vi "Minimize Polymer.vi"(8 "Error In":errorcluster, 11 "Unreacted Polymer":string) -> (0 "Error Out":errorcluster, 1 "Size of Redux Polymer":i32, 2 "Redux Polymer":string, 3 "Redux Element":string)   [LabVIEW 2019]
doc: "Produce the smallest polymer possible by removing a single element, then reacting the polymer as normal."
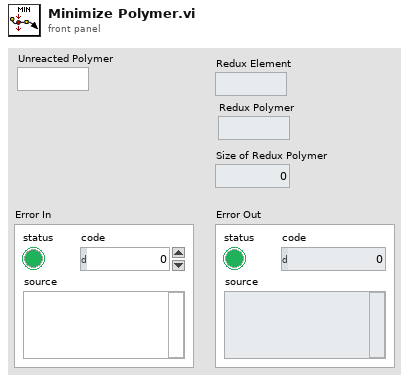
[diagram p1: front panel]
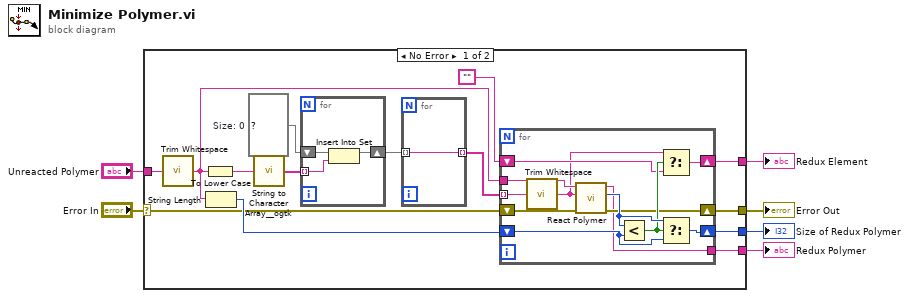
[diagram p0: block diagram]
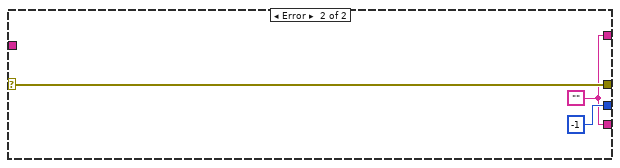
[diagram p2: hidden frame]
diagram:
  n1 = case shown="No Error" "Error In" {
    selector: "Error In" -> [w13 w38]
    tunnel: [w20 -1 ("Size of Polymer")] -> w6
    tunnel: [w19 w37] -> w5
    tunnel: "Unreacted Polymer" -> [w11 _]
    tunnel: [w12 w38] -> w2
    tunnel: [w7 w37] -> w1
    frame No Error {
      w16 = set{string} {}  # Size: 0
      n2 = call <vilib>:"Trim Whitespace.vi"("string"=w11) -> ("trimmed string"=w10:string)  [unwired: 1 in]
      n3 = To Lower Case(string=w10) -> (all lower case string=w14:string)
      n4 = String Length(string=w10) -> (length=w17:i32)
      n5 = call <userlib>:"String to Character Array__ogtk.vi"("Input String"=w14) -> ("Character Array"=w15:string[])
      n6 = for {
        tunnel: w15 -> [w35] mode=indexing
        shift-right: [w34] -> w9
        shift-left: w16 -> [w36]
        n7 = Insert Into Set(10:w35, 11:w36) -> (3:w34:set{string})  [unwired: 1 out]
      }
      n8 = for {
        tunnel: [w21] -> w8 mode=indexing
        tunnel: w9 -> [w21] mode=indexing
      }
      n9 = for {
        tunnel: w10 -> [w33]
        shift-right: [w30] -> w20
        shift-left: w17 -> [w31]
        shift-right: [w27] -> w19
        shift-left: "" -> [w28]
        shift-right: [w26] -> w12
        shift-left: w13 -> [w25]
        tunnel: w8 -> [w24] mode=indexing
        tunnel: [w22] -> w7
        n10 = call <vilib>:"Trim Whitespace.vi"("string"=w24) -> ("trimmed string"=w23:string)  [unwired: 1 in]
        n11 = call "React Polymer.vi"("Error In"=w25, "Redux Element"=w23, "Unreacted Polymer"=w33) -> ("Error Out"=w26:errorcluster, "Size of Polymer"=w32:i32, "Polymer"=w22:string)  [unwired: 6 in]
        n12 = Less?(x=w32, y=w31) -> (x < y?=w29:bool)
        n13 = Select(t=w23, s=w29, f=w28) -> (s? t:f=w27:string)
        n14 = Select(t=w32, s=w29, f=w31) -> (s? t:f=w30:i32)
      }
    }
    frame Error {
      w37 = ""
    }
  }
  "Size of Redux Polymer" <- w6
  "Redux Element" <- w5
  "Error Out" <- w2
  "Redux Polymer" <- w1
